vi "IOcheck.vi"(8 "error in (no error)":errorcluster, 9 "Variables State in":T1, 10 "HW CTRL Data":T2) -> (0 "error out":errorcluster, 1 "Variables State out":T1)   [LabVIEW 2014, in "SeqLoop.lvlib"]
doc: "Detecta el estado de las variables lógicas en función entradas digitales."
uses:
  SeqLoop.lvlib
  TypeDefs/HW CTRL Data.ctl
  TypeDefs/Variables State.ctl
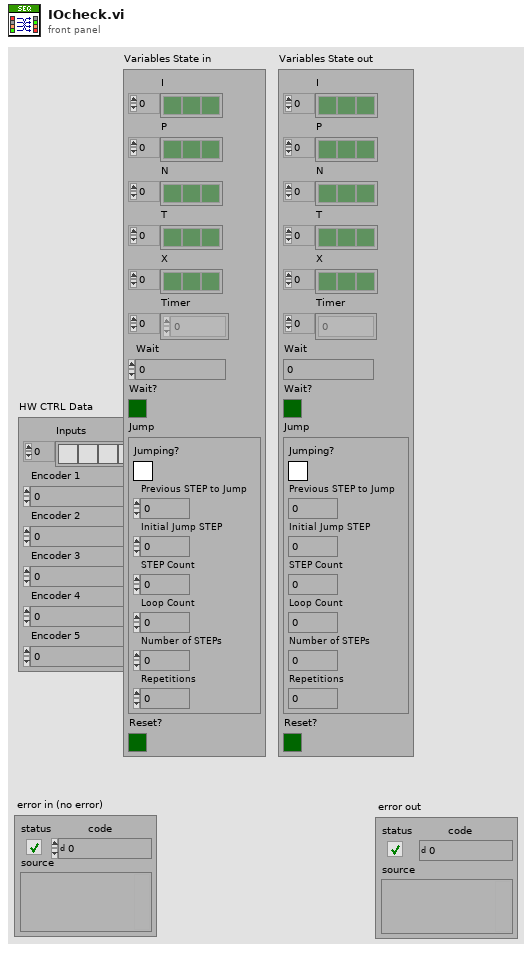
[diagram p1: front panel]
types:
  T1 = typedef "SeqLoop.lvlib/Variables State.ctl" = cluster{"I":bool[], "P":bool[], "N":bool[], "T":bool[], "X":bool[], "Timer":u32[], "Wait":u32, "Wait?":bool, "Jump":cluster{"Jumping?":bool, "Previous STEP to Jump":u32, "Initial Jump STEP":u32, "STEP Count":u32, "Loop Count":u32, "Number of STEPs":u32, "Repetitions":u32}, "Reset?":bool}
  T2 = typedef "SeqLoop.lvlib/HW CTRL Data.ctl" = cluster{"Inputs":bool[], "Encoder 1":sgl, "Encoder 2":sgl, "Encoder 3":sgl, "Encoder 4":sgl, "Encoder 5":sgl}
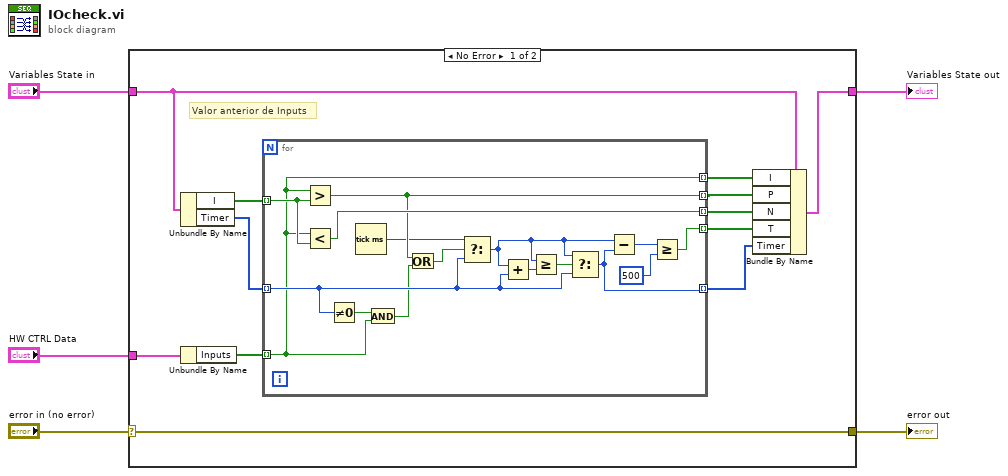
[diagram p0: block diagram]
diagram:
  n1 = case shown="No Error" "error in (no error)" {
    selector: "error in (no error)" -> [w14 w34]
    tunnel: "Variables State in" -> [w12 w35]
    tunnel: [w17 w35] -> w4
    tunnel: [w14 w34] -> w2
    tunnel: "HW CTRL Data" -> [w13 _]
    frame No Error {
      # "Valor anterior de Inputs"
      n2 = Unbundle By Name(w12) -> ("I"=w7:bool[], "Timer"=w6:u32[])
      n3 = Unbundle By Name(w13) -> ("Inputs"=w16:bool[])
      n4 = for {
        tunnel: w16 -> [w21] mode=indexing
        tunnel: [w21] -> w8 mode=indexing
        tunnel: [w26] -> w9 mode=indexing
        tunnel: w7 -> [w33] mode=indexing
        tunnel: [w32] -> w10 mode=indexing
        tunnel: w6 -> [w22] mode=indexing
        tunnel: [w27] -> w11 mode=indexing
        tunnel: [w18] -> w15 mode=indexing
        n5 = Greater?(x=w21, y=w33) -> (0:w26:bool)
        n6 = Less?(x=w21, y=w33) -> (x < y?=w32:bool)
        n7 = Not Equal To 0?(x=w22) -> (x != 0?=w19:bool)
        n8 = Tick Count (ms)() -> (millisecond timer value=w24:u32)
        n9 = And(x=w19, y=w21) -> (x .and. y?=w20:bool)
        n10 = Or(x=w26, y=w20) -> (x .or. y?=w25:bool)
        n11 = Select(t=w24, s=w25, f=w22) -> (s? t:f=w23:u32)
        n12 = Add(x=w23, y=w22) -> (x+y=w29:u32)
        n13 = Greater Or Equal?(x=w23, y=w29) -> (x >= y?=w28:bool)
        n14 = Select(t=w23, s=w28, f=w22) -> (s? t:f=w18:u32)
        n15 = Subtract(x=w23, y=w18) -> (x-y=w30:u32)
        n16 = Greater Or Equal?(x=w30, y=u32 500) -> (x >= y?=w27:bool)
      }
      n17 = Bundle By Name(cluster=w12, "I"=w8, "P"=w9, "N"=w10, "T"=w11, "Timer"=w15) -> (w17:T1)
    }
    frame Error {
    }
  }
  "Variables State out" <- w4
  "error out" <- w2
